vi "progress bar.vi"(0 "n":i32=1 min=1 step=1, 11 "weight (0-100)":dbl min=0.0 max=100.0 format="%#_13g") -> ()   [LabVIEW 2010, in "util.lvlib"]
uses:
  util.lvlib
  progress bar GV.vi
panel:
  in  "Fehler (Eingang, kein Fehler)":errorcluster
  out "Fehler (Ausgang)":errorcluster
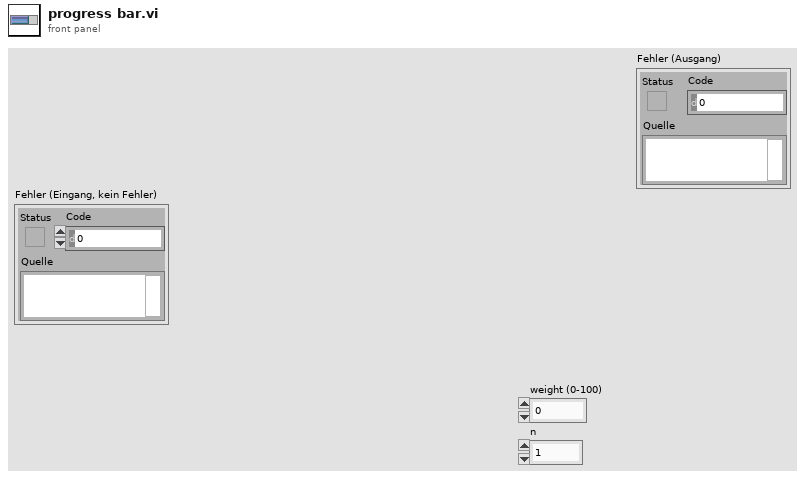
[diagram p1: front panel]
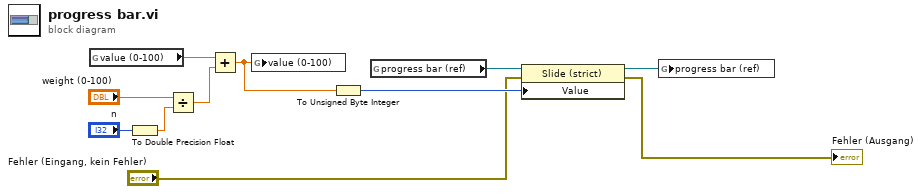
[diagram p0: block diagram]
diagram:
  n1 = global read "progress bar GV.vi" "value (0-100)"() -> (w5:dbl)
  n2 = To Double Precision Float(number="n") -> (double precision float=w6:dbl)
  n3 = Divide(x="weight (0-100)", y=w6) -> (x/y=w4:dbl)
  n4 = Add(x=w5, y=w4) -> (x+y=w3:dbl)
  n5 = global write "progress bar GV.vi" "value (0-100)"(w3) -> ()
  n6 = To Unsigned Byte Integer(number=w3) -> (unsigned 8bit integer=w8:u8)
  n7 = global read "progress bar GV.vi" "progress bar (ref)"() -> (w9:refnum<vi>)
  n8 = property on="Eigenschaftsknoten" class="Slide (strict)"(reference=w9, error in="Fehler (Eingang, kein Fehler)", "Value"=w8) -> (reference out=w10:refnum<vi>, error out=→"Fehler (Ausgang)":errorcluster)
  n9 = global write "progress bar GV.vi" "progress bar (ref)"(w10) -> ()
